vi "fluke_temp_log.vi"() -> ()   [LabVIEW 2010]
doc: "The Read Caliper VI reads data from Fowler calipers... 4800 baud, 7Bit, parity 2. Reads 5 bits and exports the resulting number. Calipers must be plugged into Com1"
uses:
  <vilib>/Instr/_visa.llb/VISA Configure Serial Port (Serial Instr).vi
panel:
  in  "bytes2read":u32
  out "String":string
  out "Numeric":u32
  out "error out":errorcluster
  in  "Parity":i8
  in  "Data Bit":i8=8
  in  "resource name":refnum<visa-resource-name>="COM2"
  in  "baud rate (9600)":u32=9600
  in  "error in (no error)":errorcluster
  # "choose appropriate port"
  # "Read Requested Bytes from Serial Port.\nThe VI will wait for the requested bytes to\nexist in the buffer.  Note in the Windows\nand Sun version, the VI initially resets the port,\nvoiding preexisitng data.  The Macintosh version\nsaves existing data in the buffer."
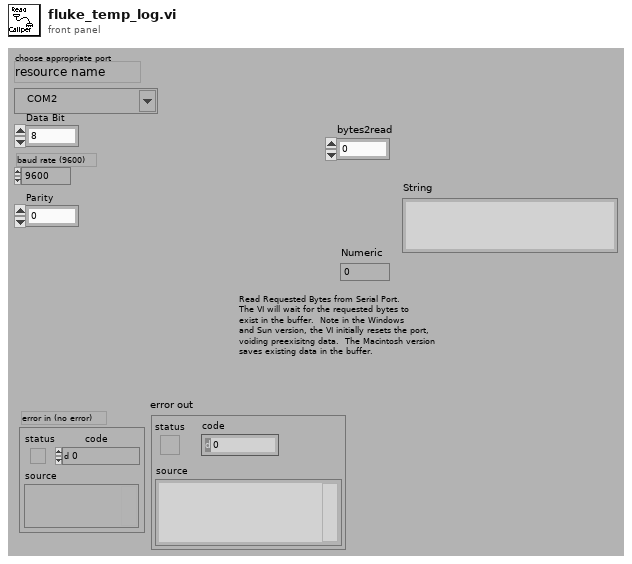
[diagram p1: front panel]
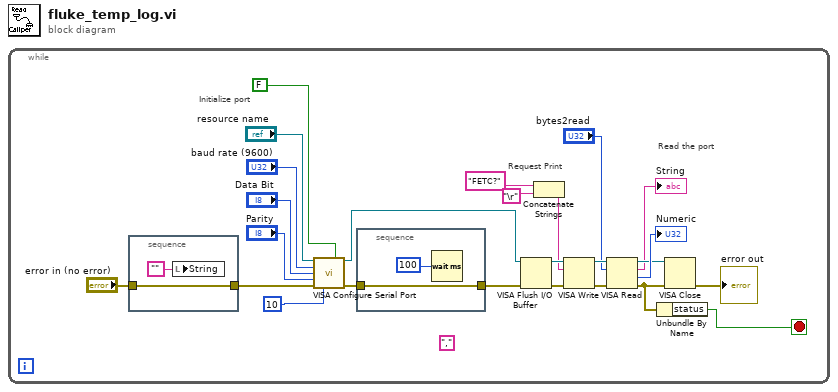
[diagram p0: block diagram]
diagram:
  n1 = while {
    stop <- w4 stop-if-true
    (unwired) ","
    # "Read the port"
    # "Request Print"
    # "Initialize port"
    n2 = stacked-sequence {
      tunnel: "error in (no error)" -> [w27]
      tunnel: [w27] -> w11
      frame #0 {
        n3 = local write "String"("") -> ()
      }
    }
    n4 = call-poly "VISA Configure Serial Port"("VISA resource name"="resource name", "Enable Termination\nChar (T)"=FALSE, "baud rate (9600)"="baud rate (9600)", "data bits (8)"="Data Bit", "parity (0:none)"="Parity", "error in (no error)"=w11, "stop bits (10: 1 bit)"=10) -> ("VISA resource name out"=w24:refnum<visa-resource-name>, "error out"=w23:errorcluster)  [unwired: 7 in]
    n5 = stacked-sequence {
      tunnel: w23 -> [w29]
      tunnel: [w29] -> w25
      frame #0 {
        n6 = Wait (ms)(milliseconds to wait=100) -> ()  [unwired: 1 out]
      }
    }
    n7 = VISA Flush I/O Buffer(VISA resource name=w24, error in (no error)=w25) -> (VISA resource name out=w18:refnum<visa-resource-name>, error out=w17:errorcluster)  [unwired: 1 in]
    n8 = Concatenate Strings("FETC?", "\r") -> (w13:string)
    n9 = VISA Write(VISA resource name=w18, write buffer=w13, error in (no error)=w17) -> (VISA resource name out=w3:refnum<visa-resource-name>, error out=w1:errorcluster)  [unwired: 1 out]
    n10 = VISA Read(VISA resource name=w3, byte count="bytes2read", error in (no error)=w1) -> (VISA resource name out=w9:refnum<visa-resource-name>, read buffer=→"String":string, return count=→"Numeric":u32, error out=w8:errorcluster)
    n11 = Unbundle By Name(w8) -> ("status"=w4:bool)
    n12 = VISA Close(VISA resource name=w9, error in (no error)=w8) -> (error out=→"error out":errorcluster)
  }
